vi "SET_play.vi"() -> ()   [LabVIEW 2018]
uses:
  Ctrl/SET_1111.ctl
  Ctrl/SET_1112.ctl
  Ctrl/SET_1113.ctl
  Ctrl/SET_1121.ctl
  Ctrl/SET_1122.ctl
  Ctrl/SET_1123.ctl
  Ctrl/SET_1131.ctl
  Ctrl/SET_1132.ctl
  Ctrl/SET_1133.ctl
  Ctrl/SET_1211.ctl
  Ctrl/SET_1212.ctl
  Ctrl/SET_1213.ctl
  Ctrl/SET_1221.ctl
  Ctrl/SET_1222.ctl
  Ctrl/SET_1223.ctl
  Ctrl/SET_1231.ctl
  Ctrl/SET_1232.ctl
  Ctrl/SET_1233.ctl
  Ctrl/SET_1311.ctl
  Ctrl/SET_1312.ctl
  Ctrl/SET_1313.ctl
  Ctrl/SET_1321.ctl
  Ctrl/SET_1322.ctl
  Ctrl/SET_1323.ctl
  Ctrl/SET_1331.ctl
  Ctrl/SET_1332.ctl
  Ctrl/SET_1333.ctl
  Ctrl/SET_2111.ctl
  Ctrl/SET_2112.ctl
  Ctrl/SET_2113.ctl
  Ctrl/SET_2121.ctl
  Ctrl/SET_2122.ctl
  Ctrl/SET_2123.ctl
  Ctrl/SET_2131.ctl
  Ctrl/SET_2132.ctl
  Ctrl/SET_2133.ctl
  Ctrl/SET_2211.ctl
  Ctrl/SET_2212.ctl
  Ctrl/SET_2213.ctl
  Ctrl/SET_2221.ctl
  Ctrl/SET_2222.ctl
  Ctrl/SET_2223.ctl
  Ctrl/SET_2231.ctl
  Ctrl/SET_2232.ctl
  Ctrl/SET_2233.ctl
  Ctrl/SET_2311.ctl
  Ctrl/SET_2312.ctl
  Ctrl/SET_2313.ctl
  Ctrl/SET_2321.ctl
  Ctrl/SET_2322.ctl
  Ctrl/SET_2323.ctl
  Ctrl/SET_2331.ctl
  Ctrl/SET_2332.ctl
  Ctrl/SET_2333.ctl
  Ctrl/SET_3111.ctl
  Ctrl/SET_3112.ctl
  Ctrl/SET_3113.ctl
  Ctrl/SET_3121.ctl
  Ctrl/SET_3122.ctl
  Ctrl/SET_3123.ctl
  Ctrl/SET_3131.ctl
  Ctrl/SET_3132.ctl
  Ctrl/SET_3133.ctl
  Ctrl/SET_3211.ctl
  Ctrl/SET_3212.ctl
  Ctrl/SET_3213.ctl
  Ctrl/SET_3221.ctl
  Ctrl/SET_3222.ctl
  Ctrl/SET_3223.ctl
  Ctrl/SET_3231.ctl
  Ctrl/SET_3232.ctl
  Ctrl/SET_3233.ctl
  Ctrl/SET_3311.ctl
  Ctrl/SET_3312.ctl
  Ctrl/SET_3313.ctl
  Ctrl/SET_3321.ctl
  Ctrl/SET_3322.ctl
  Ctrl/SET_3323.ctl
  Ctrl/SET_3331.ctl
  Ctrl/SET_3332.ctl
  Ctrl/SET_3333.ctl
  Ctrl/Button_turn.ctl
  Ctrl/Delay_time_display.ctl
  Ctrl/Color_box.ctl
  <vilib>/Utility/miscctls.llb/LVBoundsTypeDef.ctl
  <vilib>/Utility/miscctls.llb/LVPositionTypeDef.ctl
  Ctrl/Menu.ctl
  8331993e-770e-4ab0-80c5-ef35aa114950.vi
  2b4e26d8-541c-4eaa-9e7c-42fc4059c27e.vi
panel:
  out "Hint_idx":u8
  out "Matching_idx":i32[][](array[numeric])
  out "Total_ID":i32[](array[numeric])
  out "Count_shuffle":i32=12
  out "ID_select_cards":i32[](array[numeric])
  out "idx_select_cards":i32[](array[numeric])
  out "Start_time(ms)":u32
  out "Turn":bool
  out "POS_of_cards":T1[](array[typedef])
  out "main_cards":refnum<vi>[](array[refnum])
  out "Ref_turn_btn":refnum<vi>[](array[refnum])
  out "Time_turn(ms)":u32
  out "Time_disadvantage(ms)":u32
  out "Ref_card_shuffle":refnum<vi>[](array[refnum])
  out "Tab_bounds":T2 caption="경계"
  out "Ref_card":refnum<vi>[](array[refnum])
  out "Tab_ctrl":enum32{"페이지 1", "페이지 2", "페이지 3"}(tab)
  in  "exit_program":bool
  out "num_SET":u8
  out "num_remain_cards":u8
  out "Delay_2P":T3 scale=0.0..1.0
  in  "Turn_2P":T4
  out "Delay_1P":T3 scale=0.0..1.0
  in  "Turn_1P":T4
  in  "불리언 81":T5
  in  "불리언 80":T6
  in  "불리언 79":T7
  in  "불리언 78":T8
  in  "불리언 77":T9
  in  "불리언 76":T10
  in  "불리언 75":T11
  in  "불리언 74":T12
  in  "불리언 73":T13
  in  "불리언 72":T14
  in  "불리언 71":T15
  in  "불리언 70":T16
  in  "불리언 69":T17
  in  "불리언 68":T18
  in  "불리언 67":T19
  in  "불리언 66":T20
  in  "불리언 65":T21
  in  "불리언 64":T22
  in  "불리언 63":T23
  in  "불리언 62":T24
  in  "불리언 61":T25
  in  "불리언 60":T26
  in  "불리언 59":T27
  in  "불리언 58":T28
  in  "불리언 57":T29
  in  "불리언 56":T30
  in  "불리언 55":T31
  in  "불리언 54":T32
  in  "불리언 53":T33
  in  "불리언 52":T34
  in  "불리언 51":T35
  in  "불리언 50":T36
  in  "불리언 49":T37
  in  "불리언 48":T38
  in  "불리언 47":T39
  in  "불리언 46":T40
  in  "불리언 45":T41
  in  "불리언 44":T42
  in  "불리언 43":T43
  in  "불리언 42":T44
  in  "불리언 41":T45
  in  "불리언 40":T46
  in  "불리언 39":T47
  in  "불리언 38":T48
  in  "불리언 37":T49
  in  "불리언 36":T50
  in  "불리언 35":T51
  in  "불리언 34":T52
  in  "불리언 33":T53
  in  "불리언 32":T54
  in  "불리언 31":T55
  in  "불리언 30":T56
  in  "불리언 29":T57
  in  "불리언 28":T58
  in  "불리언 27":T59
  in  "불리언 26":T60
  in  "불리언 25":T61
  in  "불리언 24":T62
  in  "불리언 23":T63
  in  "불리언 22":T64
  in  "불리언 21":T65
  in  "불리언 20":T66
  in  "불리언 19":T67
  in  "불리언 18":T68
  in  "불리언 17":T69
  in  "불리언 16":T70
  in  "불리언 15":T71
  in  "불리언 14":T72
  in  "불리언 13":T73
  in  "불리언 12":T74
  in  "불리언 11":T75
  in  "불리언 10":T76
  in  "불리언 9":T77
  in  "불리언 8":T78
  in  "불리언 7":T79
  in  "불리언 6":T80
  in  "불리언 5":T81
  in  "불리언 4":T82
  in  "불리언 3":T83
  in  "불리언 2":T84
  in  "불리언":T85
  out "Color_box_1P":T86
  out "Color_box_2P":T86
  in  "Button_start":bool
  out "Score_1P":i8
  out "Score_2P":i8
  in  "Btn_hint":bool
  # "1P\nScore"
  # "2P\nScore"
  # "남은\n카드"
  # "SET\n개수"
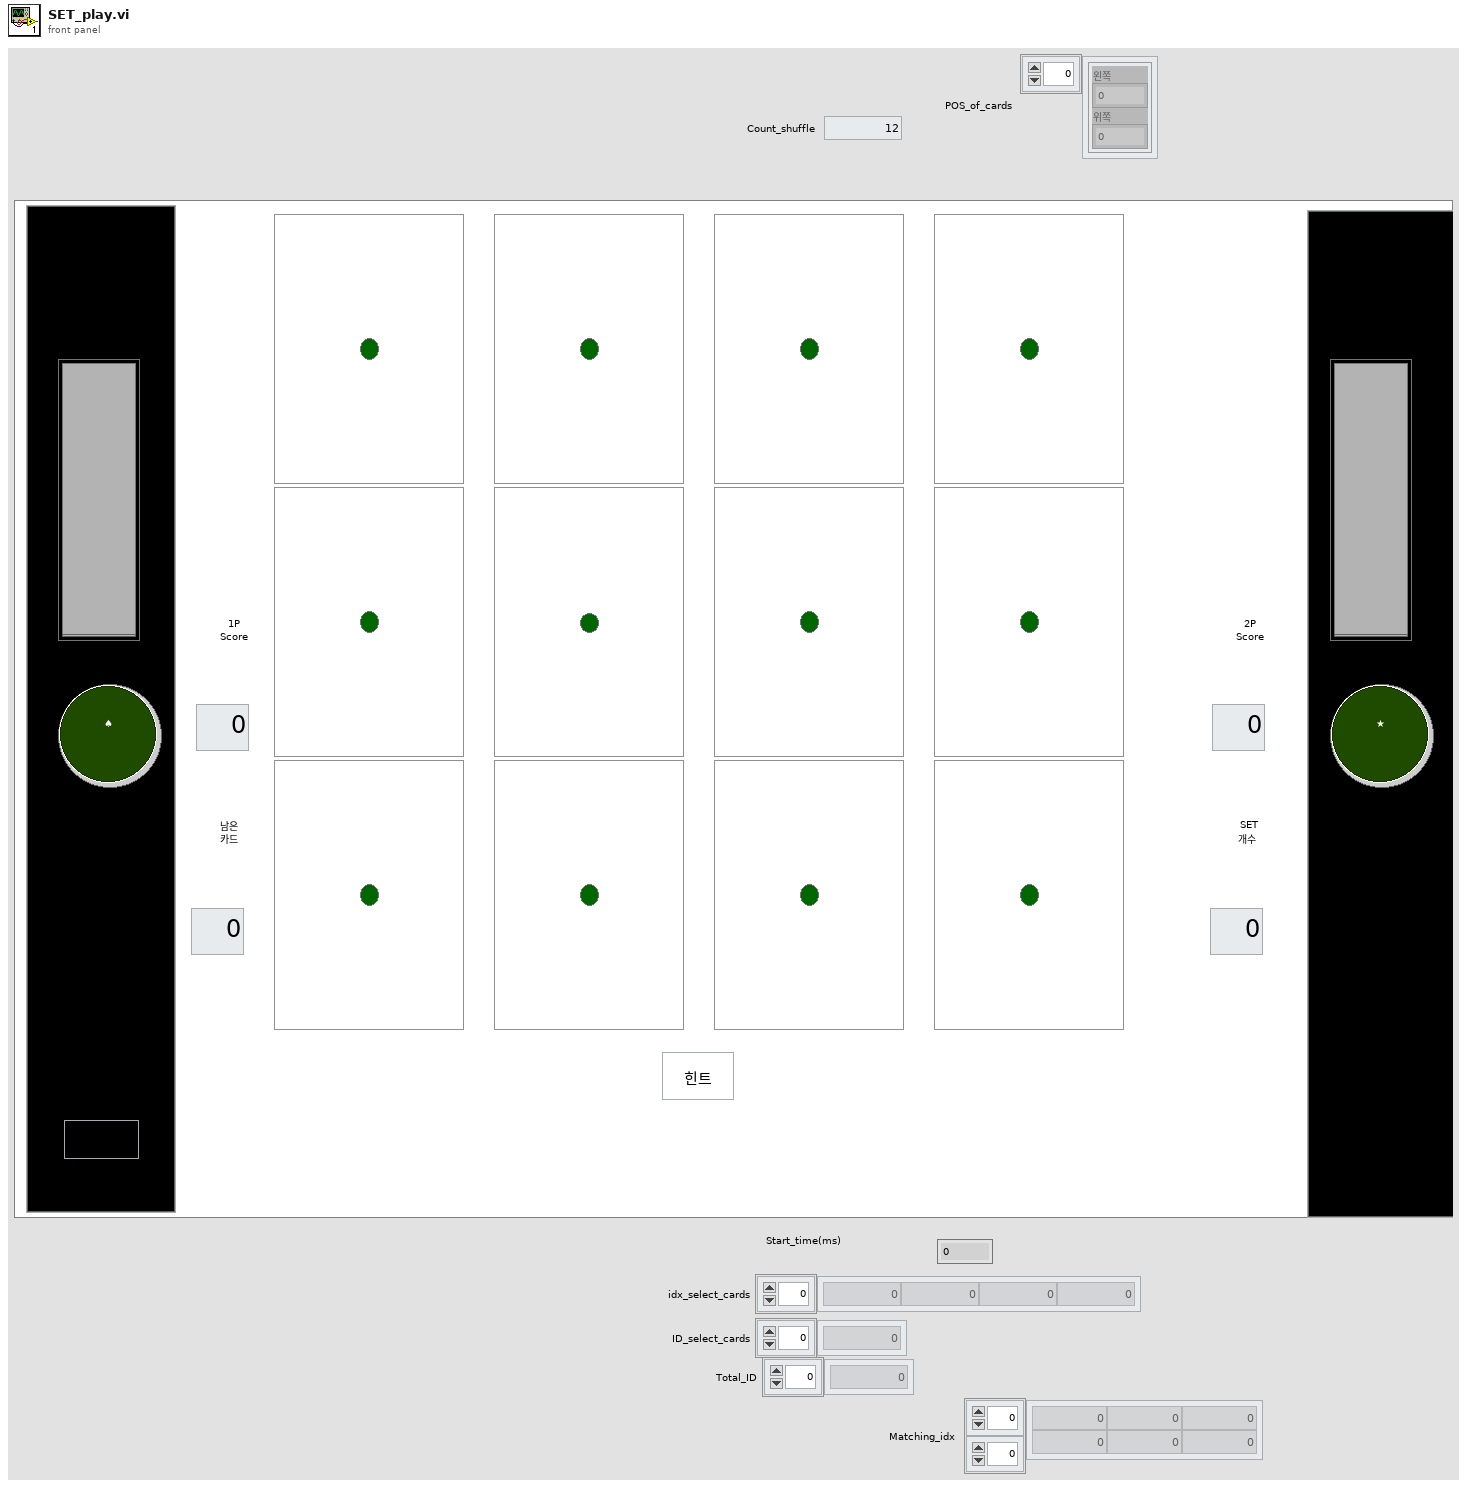
[diagram p1: front panel]
types:
  T1 = typedef "LVPositionTypeDef.ctl" = cluster{"Left":i32, "Top":i32}
  T2 = typedef "LVBoundsTypeDef.ctl" = cluster{"Width":u32, "Height":u32}
  T3 = typedef "Delay_time_display.ctl" = dbl
  T4 = typedef "Button_turn.ctl" = bool
  T5 = typedef "SET_3333.ctl" = bool
  T6 = typedef "SET_3332.ctl" = bool
  T7 = typedef "SET_3331.ctl" = bool
  T8 = typedef "SET_3323.ctl" = bool
  T9 = typedef "SET_3322.ctl" = bool
  T10 = typedef "SET_3321.ctl" = bool
  T11 = typedef "SET_3313.ctl" = bool
  T12 = typedef "SET_3312.ctl" = bool
  T13 = typedef "SET_3311.ctl" = bool
  T14 = typedef "SET_3233.ctl" = bool
  T15 = typedef "SET_3232.ctl" = bool
  T16 = typedef "SET_3231.ctl" = bool
  T17 = typedef "SET_3223.ctl" = bool
  T18 = typedef "SET_3222.ctl" = bool
  T19 = typedef "SET_3221.ctl" = bool
  T20 = typedef "SET_3213.ctl" = bool
  T21 = typedef "SET_3212.ctl" = bool
  T22 = typedef "SET_3211.ctl" = bool
  T23 = typedef "SET_3133.ctl" = bool
  T24 = typedef "SET_3132.ctl" = bool
  T25 = typedef "SET_3131.ctl" = bool
  T26 = typedef "SET_3123.ctl" = bool
  T27 = typedef "SET_3122.ctl" = bool
  T28 = typedef "SET_3121.ctl" = bool
  T29 = typedef "SET_3113.ctl" = bool
  T30 = typedef "SET_3112.ctl" = bool
  T31 = typedef "SET_3111.ctl" = bool
  T32 = typedef "SET_2333.ctl" = bool
  T33 = typedef "SET_2332.ctl" = bool
  T34 = typedef "SET_2331.ctl" = bool
  T35 = typedef "SET_2323.ctl" = bool
  T36 = typedef "SET_2322.ctl" = bool
  T37 = typedef "SET_2321.ctl" = bool
  T38 = typedef "SET_2313.ctl" = bool
  T39 = typedef "SET_2312.ctl" = bool
  T40 = typedef "SET_2311.ctl" = bool
  T41 = typedef "SET_2233.ctl" = bool
  T42 = typedef "SET_2232.ctl" = bool
  T43 = typedef "SET_2231.ctl" = bool
  T44 = typedef "SET_2223.ctl" = bool
  T45 = typedef "SET_2222.ctl" = bool
  T46 = typedef "SET_2221.ctl" = bool
  T47 = typedef "SET_2213.ctl" = bool
  T48 = typedef "SET_2212.ctl" = bool
  T49 = typedef "SET_2211.ctl" = bool
  T50 = typedef "SET_2133.ctl" = bool
  T51 = typedef "SET_2132.ctl" = bool
  T52 = typedef "SET_2131.ctl" = bool
  T53 = typedef "SET_2123.ctl" = bool
  T54 = typedef "SET_2122.ctl" = bool
  T55 = typedef "SET_2121.ctl" = bool
  T56 = typedef "SET_2113.ctl" = bool
  T57 = typedef "SET_2112.ctl" = bool
  T58 = typedef "SET_2111.ctl" = bool
  T59 = typedef "SET_1333.ctl" = bool
  T60 = typedef "SET_1332.ctl" = bool
  T61 = typedef "SET_1331.ctl" = bool
  T62 = typedef "SET_1323.ctl" = bool
  T63 = typedef "SET_1322.ctl" = bool
  T64 = typedef "SET_1321.ctl" = bool
  T65 = typedef "SET_1313.ctl" = bool
  T66 = typedef "SET_1312.ctl" = bool
  T67 = typedef "SET_1311.ctl" = bool
  T68 = typedef "SET_1233.ctl" = bool
  T69 = typedef "SET_1232.ctl" = bool
  T70 = typedef "SET_1231.ctl" = bool
  T71 = typedef "SET_1223.ctl" = bool
  T72 = typedef "SET_1222.ctl" = bool
  T73 = typedef "SET_1221.ctl" = bool
  T74 = typedef "SET_1213.ctl" = bool
  T75 = typedef "SET_1212.ctl" = bool
  T76 = typedef "SET_1211.ctl" = bool
  T77 = typedef "SET_1133.ctl" = bool
  T78 = typedef "SET_1132.ctl" = bool
  T79 = typedef "SET_1131.ctl" = bool
  T80 = typedef "SET_1123.ctl" = bool
  T81 = typedef "SET_1122.ctl" = bool
  T82 = typedef "SET_1121.ctl" = bool
  T83 = typedef "SET_1113.ctl" = bool
  T84 = typedef "SET_1112.ctl" = bool
  T85 = typedef "SET_1111.ctl" = bool
  T86 = typedef "Color_box.ctl" = u32
  T87 = typedef "Menu.ctl" = enum16{"Select turn", "Initialization", "Make variable_1", "Make variable_2", "Ready game", "Choose cards", "Penalty", "Card matching", "Card checking", "Finish game", "Shuffle cards", "Hint"}
  T88 = enum8{"Enabled", "Disabled", "Disabled and Grayed Out"}
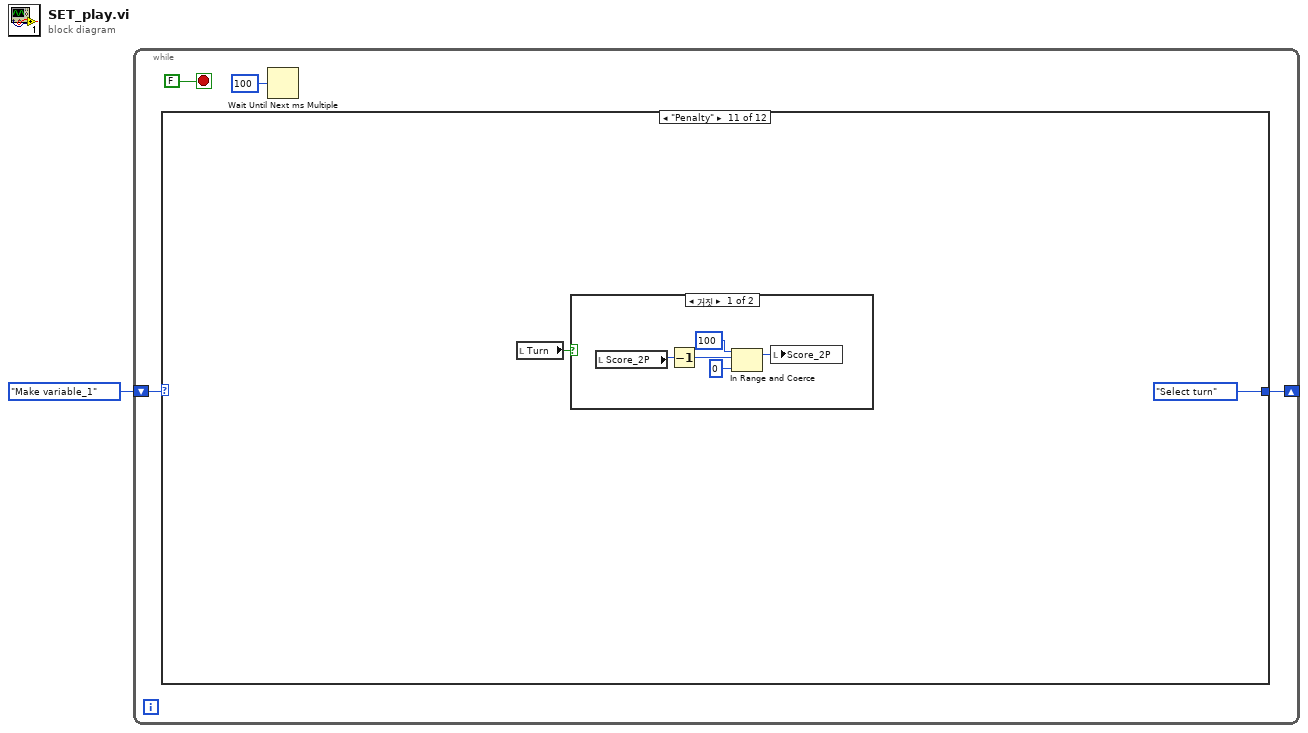
[diagram p0: block diagram]
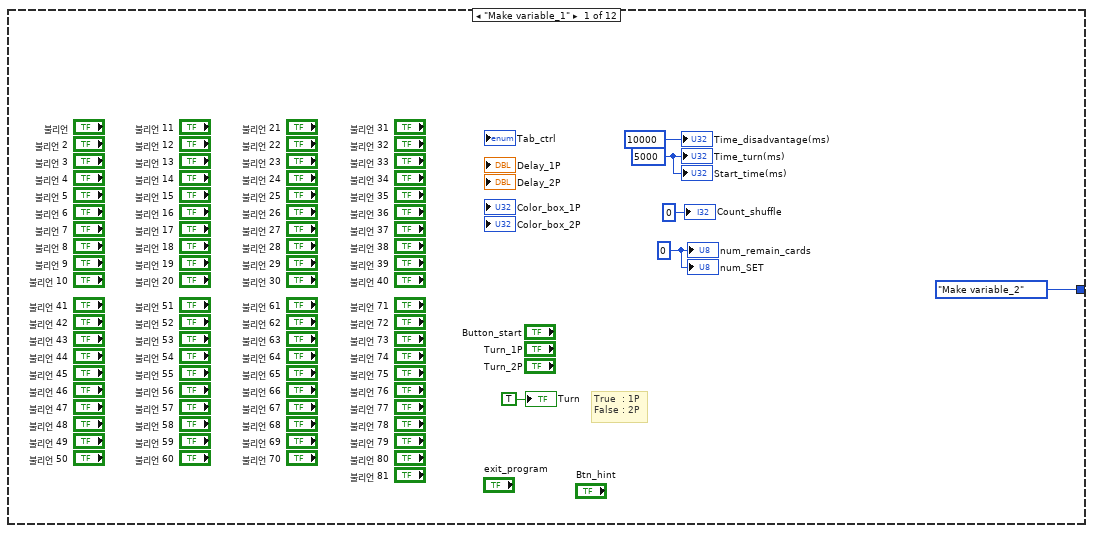
[diagram p2: hidden frame]
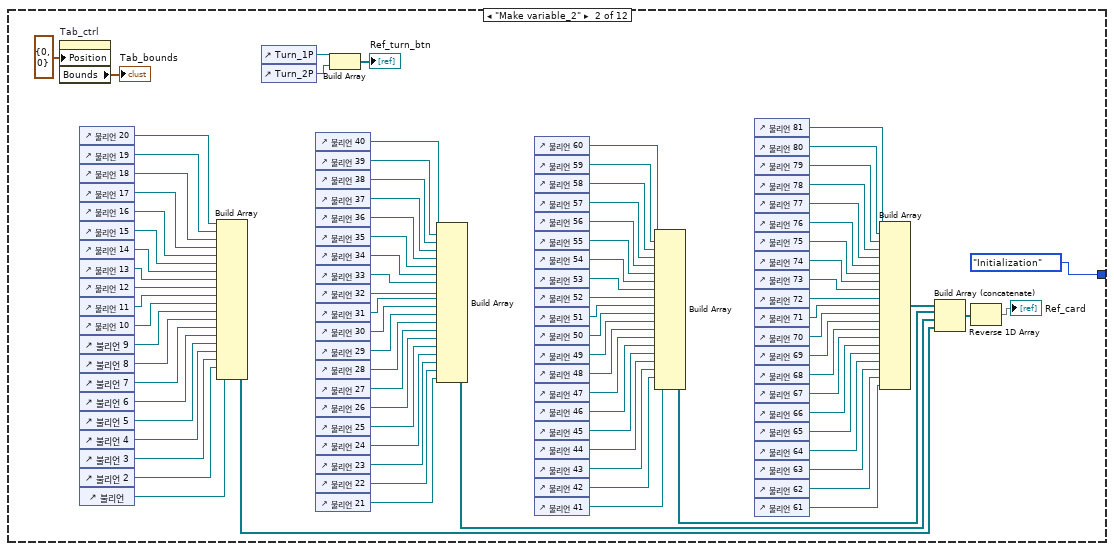
[diagram p3: hidden frame]
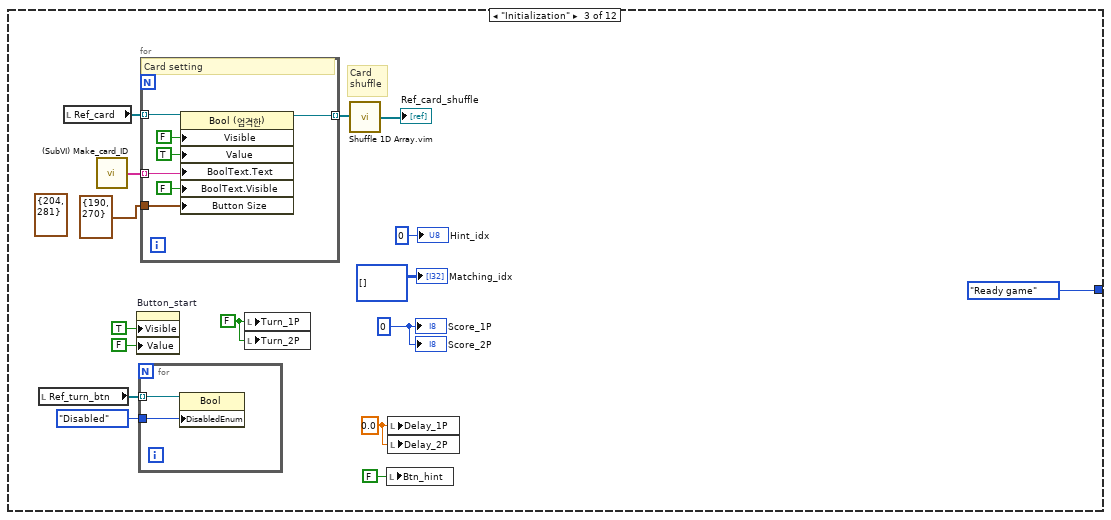
[diagram p4: hidden frame]
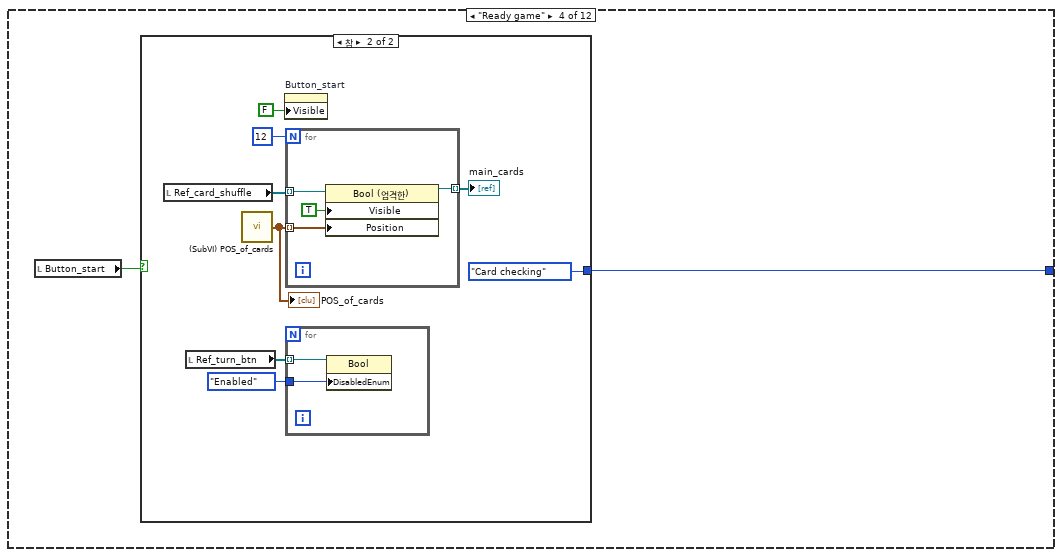
[diagram p5: hidden frame]
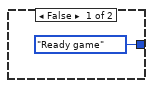
[diagram p6: hidden frame]
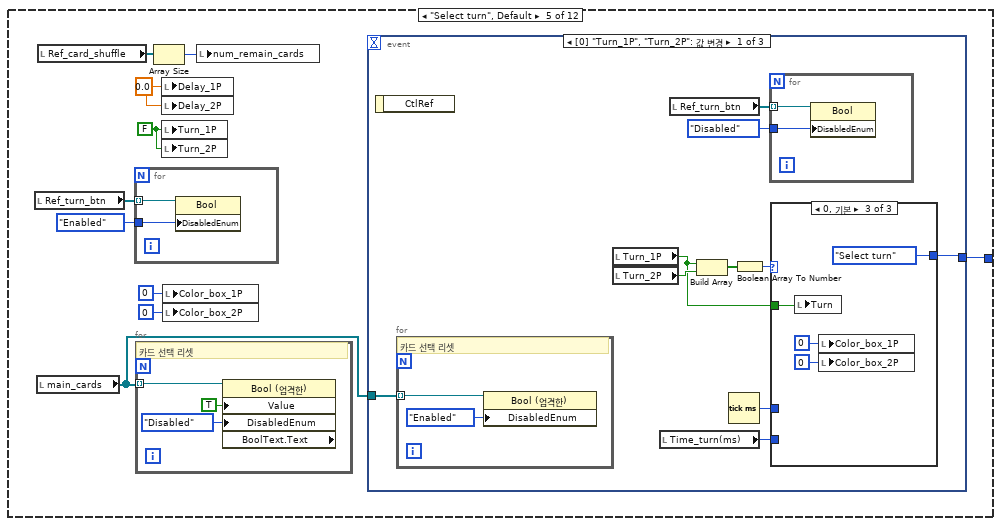
[diagram p7: hidden frame]
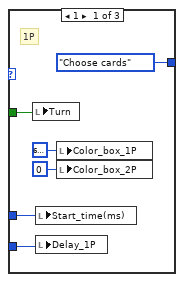
[diagram p8: hidden frame]
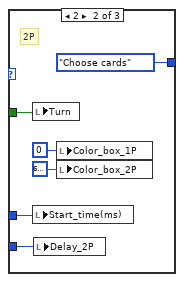
[diagram p9: hidden frame]
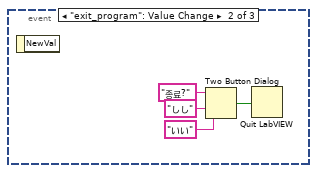
[diagram p10: hidden frame]
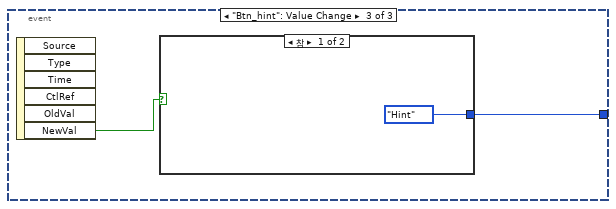
[diagram p11: hidden frame]
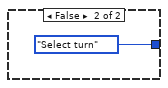
[diagram p12: hidden frame]
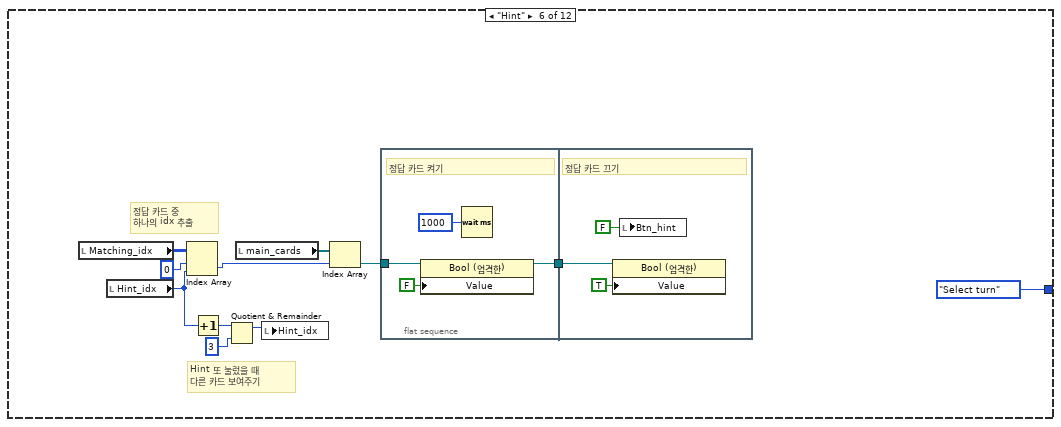
[diagram p13: hidden frame]
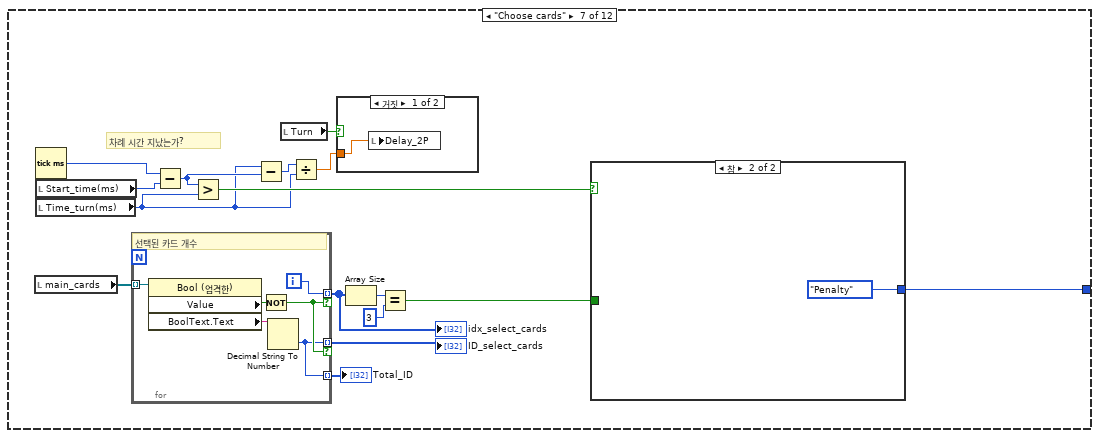
[diagram p14: hidden frame]
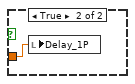
[diagram p15: hidden frame]
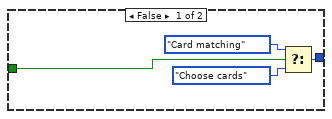
[diagram p16: hidden frame]
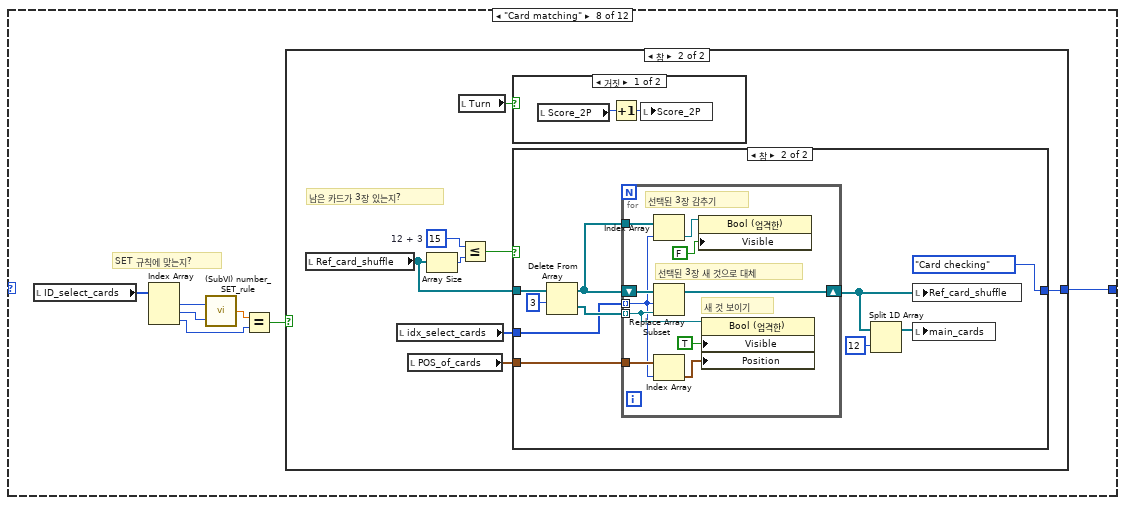
[diagram p17: hidden frame]
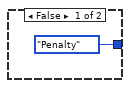
[diagram p18: hidden frame]
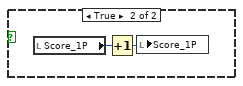
[diagram p19: hidden frame]
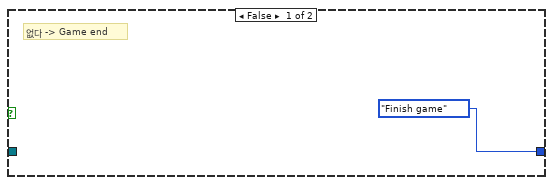
[diagram p20: hidden frame]
diagram:
  n1 = while {
    shift-right: [w3] -> _
    shift-left: Menu."Make variable_1" ("열거형") -> [w4]
    stop <- FALSE stop-if-true
    n2 = case shown="\"Penalty\"" w4 {
      tunnel: [Menu."Make variable_2" ("열거형") Menu."Initialization" ("열거형") Menu."Ready game" ("열거형") w131 w156 Menu."Select turn" ("열거형") w225 w247 w294 w306 Menu."Select turn" ("열거형") Menu."Make variable_1" ("열거형")] -> w3
      frame "Make variable_1" {
        w6 = u8 0 ("num_remain_cards")
        w8 = u32 5000 ("Time_turn(ms)")
        # "True  : 1P\nFalse : 2P"
        "Time_disadvantage(ms)" <- u32 10000 ("Time_disadvantage")
        "Time_turn(ms)" <- w8
        "Turn" <- TRUE ("Turn")
        "Start_time(ms)" <- w8
        "Count_shuffle" <- 0 ("Count_shuffle")
        "num_remain_cards" <- w6
        "num_SET" <- w6
      }
      frame "Make variable_2" {
        n3 = property on="Tab_ctrl" class="TabCtl (엄격한)"("Position"=T1 {"Left"=0, "Top"=0} ("위치")) -> ("Bounds"=→"Tab_bounds":T2)  [unwired: 2 in, 2 out]
        n4 = control-ref of="불리언 20"() -> (w25:refnum<vi>)
        n5 = control-ref of="불리언 19"() -> (w26:refnum<vi>)
        n6 = control-ref of="불리언 18"() -> (w27:refnum<vi>)
        n7 = control-ref of="불리언 17"() -> (w28:refnum<vi>)
        n8 = control-ref of="불리언 16"() -> (w29:refnum<vi>)
        n9 = control-ref of="불리언 15"() -> (w30:refnum<vi>)
        n10 = control-ref of="불리언 14"() -> (w31:refnum<vi>)
        n11 = control-ref of="불리언 13"() -> (w32:refnum<vi>)
        n12 = control-ref of="불리언 12"() -> (w33:refnum<vi>)
        n13 = control-ref of="불리언 11"() -> (w34:refnum<vi>)
        n14 = control-ref of="불리언 10"() -> (w35:refnum<vi>)
        n15 = control-ref of="불리언 9"() -> (w36:refnum<vi>)
        n16 = control-ref of="불리언 8"() -> (w37:refnum<vi>)
        n17 = control-ref of="불리언 7"() -> (w38:refnum<vi>)
        n18 = control-ref of="불리언 6"() -> (w39:refnum<vi>)
        n19 = control-ref of="불리언 5"() -> (w40:refnum<vi>)
        n20 = control-ref of="불리언 4"() -> (w41:refnum<vi>)
        n21 = control-ref of="불리언 3"() -> (w42:refnum<vi>)
        n22 = control-ref of="불리언 2"() -> (w43:refnum<vi>)
        n23 = control-ref of="불리언"() -> (w44:refnum<vi>)
        n24 = Build Array(w25, w26, w27, w28, w29, w30, w31, w32, w33, w34, w35, w36, w37, w38, w39, w40, w41, w42, w43, w44) -> (w20:refnum<vi>[])
        n25 = control-ref of="Turn_1P"() -> (w13:refnum<vi>)
        n26 = control-ref of="Turn_2P"() -> (w14:refnum<vi>)
        n27 = control-ref of="불리언 40"() -> (w45:refnum<vi>)
        n28 = control-ref of="불리언 39"() -> (w46:refnum<vi>)
        n29 = control-ref of="불리언 38"() -> (w47:refnum<vi>)
        n30 = control-ref of="불리언 37"() -> (w48:refnum<vi>)
        n31 = control-ref of="불리언 36"() -> (w49:refnum<vi>)
        n32 = control-ref of="불리언 35"() -> (w50:refnum<vi>)
        n33 = control-ref of="불리언 34"() -> (w51:refnum<vi>)
        n34 = control-ref of="불리언 33"() -> (w52:refnum<vi>)
        n35 = control-ref of="불리언 32"() -> (w53:refnum<vi>)
        n36 = control-ref of="불리언 31"() -> (w54:refnum<vi>)
        n37 = control-ref of="불리언 30"() -> (w55:refnum<vi>)
        n38 = control-ref of="불리언 29"() -> (w56:refnum<vi>)
        n39 = control-ref of="불리언 28"() -> (w57:refnum<vi>)
        n40 = control-ref of="불리언 27"() -> (w58:refnum<vi>)
        n41 = control-ref of="불리언 26"() -> (w59:refnum<vi>)
        n42 = control-ref of="불리언 25"() -> (w60:refnum<vi>)
        n43 = control-ref of="불리언 24"() -> (w61:refnum<vi>)
        n44 = control-ref of="불리언 23"() -> (w62:refnum<vi>)
        n45 = control-ref of="불리언 22"() -> (w63:refnum<vi>)
        n46 = control-ref of="불리언 21"() -> (w64:refnum<vi>)
        n47 = Build Array(w13, w14) -> (→"Ref_turn_btn":refnum<vi>[])
        n48 = Build Array(w45, w46, w47, w48, w49, w50, w51, w52, w53, w54, w55, w56, w57, w58, w59, w60, w61, w62, w63, w64) -> (w21:refnum<vi>[])
        n49 = control-ref of="불리언 60"() -> (w65:refnum<vi>)
        n50 = control-ref of="불리언 59"() -> (w66:refnum<vi>)
        n51 = control-ref of="불리언 58"() -> (w67:refnum<vi>)
        n52 = control-ref of="불리언 57"() -> (w68:refnum<vi>)
        n53 = control-ref of="불리언 56"() -> (w69:refnum<vi>)
        n54 = control-ref of="불리언 55"() -> (w70:refnum<vi>)
        n55 = control-ref of="불리언 54"() -> (w71:refnum<vi>)
        n56 = control-ref of="불리언 53"() -> (w72:refnum<vi>)
        n57 = control-ref of="불리언 52"() -> (w73:refnum<vi>)
        n58 = control-ref of="불리언 51"() -> (w74:refnum<vi>)
        n59 = control-ref of="불리언 50"() -> (w75:refnum<vi>)
        n60 = control-ref of="불리언 49"() -> (w76:refnum<vi>)
        n61 = control-ref of="불리언 48"() -> (w77:refnum<vi>)
        n62 = control-ref of="불리언 47"() -> (w78:refnum<vi>)
        n63 = control-ref of="불리언 46"() -> (w79:refnum<vi>)
        n64 = control-ref of="불리언 45"() -> (w80:refnum<vi>)
        n65 = control-ref of="불리언 44"() -> (w81:refnum<vi>)
        n66 = control-ref of="불리언 43"() -> (w82:refnum<vi>)
        n67 = control-ref of="불리언 42"() -> (w83:refnum<vi>)
        n68 = control-ref of="불리언 41"() -> (w84:refnum<vi>)
        n69 = Build Array(w65, w66, w67, w68, w69, w70, w71, w72, w73, w74, w75, w76, w77, w78, w79, w80, w81, w82, w83, w84) -> (w22:refnum<vi>[])
        n70 = control-ref of="불리언 81"() -> (w24:refnum<vi>)
        n71 = control-ref of="불리언 80"() -> (w85:refnum<vi>)
        n72 = control-ref of="불리언 79"() -> (w86:refnum<vi>)
        n73 = control-ref of="불리언 78"() -> (w87:refnum<vi>)
        n74 = control-ref of="불리언 77"() -> (w88:refnum<vi>)
        n75 = control-ref of="불리언 76"() -> (w89:refnum<vi>)
        n76 = control-ref of="불리언 75"() -> (w90:refnum<vi>)
        n77 = control-ref of="불리언 74"() -> (w91:refnum<vi>)
        n78 = control-ref of="불리언 73"() -> (w92:refnum<vi>)
        n79 = control-ref of="불리언 72"() -> (w93:refnum<vi>)
        n80 = control-ref of="불리언 71"() -> (w94:refnum<vi>)
        n81 = control-ref of="불리언 70"() -> (w95:refnum<vi>)
        n82 = control-ref of="불리언 69"() -> (w96:refnum<vi>)
        n83 = control-ref of="불리언 68"() -> (w97:refnum<vi>)
        n84 = control-ref of="불리언 67"() -> (w98:refnum<vi>)
        n85 = control-ref of="불리언 66"() -> (w99:refnum<vi>)
        n86 = control-ref of="불리언 65"() -> (w100:refnum<vi>)
        n87 = control-ref of="불리언 64"() -> (w101:refnum<vi>)
        n88 = control-ref of="불리언 63"() -> (w102:refnum<vi>)
        n89 = control-ref of="불리언 62"() -> (w103:refnum<vi>)
        n90 = control-ref of="불리언 61"() -> (w104:refnum<vi>)
        n91 = Build Array(w24, w85, w86, w87, w88, w89, w90, w91, w92, w93, w94, w95, w96, w97, w98, w99, w100, w101, w102, w103, w104) -> (w23:refnum<vi>[])
        n92 = Build Array (concatenate)(w23, w22, w21, w20) -> (w19:refnum<vi>[])
        n93 = Reverse 1D Array(array=w19) -> (reversed array=→"Ref_card":refnum<vi>[])
      }
      frame "Initialization" {
        w105 = i8 0 ("Score_1P")
        (unwired) T2 {"Width"=204, "Height"=281} ("버튼 크기")
        w110 = T3 0.0 ("Delay_1P")
        w113 = T4 FALSE ("Turn_1P")
        # "Card \nshuffle"
        n94 = local read "Ref_turn_btn"() -> (w114:refnum<vi>[])
        n95 = local read "Ref_card"() -> (w120:refnum<vi>[])
        n96 = call "(SubVI) Make_card_ID.vi"() -> ("Card_ID"=w119:string[])
        n97 = property on="Button_start" class="Bool (엄격한)"("Visible"=TRUE ("보이기"), "Value"=FALSE ("Button_start")) -> ()  [unwired: 2 in, 2 out]
        n98 = for {
          tunnel: T88."Disabled" ("비활성화") -> [w122]
          tunnel: w114 -> [w121] mode=indexing
          n99 = property class="Bool"(reference=w121, "DisabledEnum"=w122) -> ()  [unwired: 1 in, 2 out]
        }
        n100 = for {
          tunnel: w120 -> [w129] mode=indexing
          tunnel: w119 -> [w125] mode=indexing
          tunnel: [w124] -> w118 mode=indexing
          tunnel: T2 {"Width"=190, "Height"=270} ("버튼 크기") -> [w123]
          # "Card setting"
          n101 = property class="Bool (엄격한)"(reference=w129, "Visible"=FALSE ("보이기"), "Value"=T85 TRUE ("값"), "BoolText.Text"=w125, "BoolText.Visible"=FALSE ("불리언 텍스트.보이기"), "Button Size"=w123) -> (reference out=w124:refnum<vi>)  [unwired: 1 in, 1 out]
        }
        n102 = local write "Turn_1P"(w113) -> ()
        n103 = local write "Turn_2P"(w113) -> ()
        n104 = call "Shuffle 1D Array.vim"("array"=w118) -> ("shuffled array"=→"Ref_card_shuffle":refnum<vi>[])  [unwired: 4 in]
        n105 = local write "Btn_hint"(FALSE ("Btn_hint")) -> ()
        n106 = local write "Delay_1P"(w110) -> ()
        n107 = local write "Delay_2P"(w110) -> ()
        "Score_1P" <- w105
        "Score_2P" <- w105
        "Matching_idx" <- i32[][] [] ("Matching_idx")
        "Hint_idx" <- u8 0 ("Hint_idx")
      }
      frame "Ready game" {
        n108 = local read "Button_start"() -> (w130:bool)
        n109 = case shown="참" w130 {
          tunnel: [Menu."Ready game" ("열거형") Menu."Card checking" ("열거형")] -> w131
          frame False {
          }
          frame True {
            n110 = local read "Ref_card_shuffle"() -> (w138:refnum<vi>[])
            n111 = local read "Ref_turn_btn"() -> (w136:refnum<vi>[])
            n112 = call "(SubVI) POS_of_cards.vi"() -> ("POS_of_cards"=w139:T1[])
            "POS_of_cards" <- w139
            n113 = property on="Button_start" class="Bool (엄격한)"("Visible"=FALSE ("보이기")) -> ()  [unwired: 2 in, 2 out]
            n114 = for {
              N: 12 -> [_]
              tunnel: w138 -> [w146] mode=indexing
              tunnel: w139 -> [w144] mode=indexing
              tunnel: [w143] -> w133 mode=indexing
              n115 = property class="Bool (엄격한)"(reference=w146, "Visible"=TRUE ("보이기"), "Position"=w144) -> (reference out=w143:refnum<vi>)  [unwired: 1 in, 1 out]
            }
            "main_cards" <- w133
            n116 = for {
              tunnel: T88."Enabled" ("비활성화") -> [w142]
              tunnel: w136 -> [w141] mode=indexing
              n117 = property class="Bool"(reference=w141, "DisabledEnum"=w142) -> ()  [unwired: 1 in, 2 out]
            }
          }
        }
      }
      frame "Select turn", Default {
        w149 = T3 0.0 ("Delay_1P")
        w150 = T4 FALSE ("Turn_1P")
        n118 = local read "Ref_turn_btn"() -> (w151:refnum<vi>[])
        n119 = local read "main_cards"() -> (w155:refnum<vi>[])
        n120 = local read "Ref_card_shuffle"() -> (w147:refnum<vi>[])
        n121 = for {
          tunnel: T88."Enabled" ("비활성화") -> [w158]
          tunnel: w151 -> [w157] mode=indexing
          n122 = property class="Bool"(reference=w157, "DisabledEnum"=w158) -> ()  [unwired: 1 in, 2 out]
        }
        n123 = for {
          tunnel: w155 -> [w160] mode=indexing
          # "카드 선택 리셋"
          n124 = property class="Bool (엄격한)" props=["Value", "DisabledEnum", "BoolText", "Text"](reference=w160, "Value"=TRUE ("보이기"), "DisabledEnum"=T88."Disabled" ("비활성화")) -> ()  [unwired: 1 in, 3 out]
        }
        n125 = Array Size(array=w147) -> (size(s)=w148:i32)
        n126 = local write "Delay_1P"(w149) -> ()
        n127 = local write "Delay_2P"(w149) -> ()
        n128 = local write "Turn_1P"(w150) -> ()
        n129 = local write "Turn_2P"(w150) -> ()
        n130 = local write "Color_box_1P"(T86 0 ("Color_box_1P")) -> ()
        n131 = local write "Color_box_2P"(T86 0 ("Color_box_2P")) -> ()
        n132 = local write "num_remain_cards"(w148) -> ()
        n133 = event shown="[0] \"Turn_1P\", \"Turn_2P\": 값 변경" {
          selector: _ -> [_ _ _]
          dyn-events: _ -> [_ _ _]
          timeout: _ -> [_ _ _]
          tunnel: [w168 _ w196] -> w156
          tunnel: w155 -> [w163 _ _]
          event Value Change {
            n134 = event-data() -> ()  [unwired: 1 in, 1 out]
            n135 = for {
              tunnel: w163 -> [w172] mode=indexing
              # "카드 선택 리셋"
              n136 = property class="Bool (엄격한)"(reference=w172, "DisabledEnum"=T88."Enabled" ("비활성화")) -> ()  [unwired: 1 in, 2 out]
            }
            n137 = local read "Turn_1P"() -> (w167:T4)
            n138 = local read "Turn_2P"() -> (w171:T4)
            n139 = local read "Time_turn(ms)"() -> (w162:u32)
            n140 = local read "Ref_turn_btn"() -> (w170:refnum<vi>[])
            n141 = Build Array(w167, w171) -> (w166:T4[])
            n142 = Tick Count (ms)() -> (millisecond timer value=w164:u32)
            n143 = Boolean Array To Number(Boolean array=w166) -> (number=w165:u32)
            n144 = for {
              tunnel: T88."Disabled" ("비활성화") -> [w191]
              tunnel: w170 -> [w190] mode=indexing
              n145 = property class="Bool"(reference=w190, "DisabledEnum"=w191) -> ()  [unwired: 1 in, 2 out]
            }
            n146 = case shown="0, 기본" w165 {
              tunnel: [Menu."Choose cards" ("열거형") Menu."Choose cards" ("열거형") Menu."Select turn" ("열거형")] -> w168
              tunnel: w167 -> [w178 w184 w188]
              tunnel: w164 -> [w175 w181 _]
              tunnel: w162 -> [w174 w180 _]
              frame 1 {
                # "1P"
                n147 = local write "Turn"(w178) -> ()
                n148 = local write "Start_time(ms)"(w175) -> ()
                n149 = local write "Delay_1P"(w174) -> ()
                n150 = local write "Color_box_1P"(T86 6618880 ("Color_box_1P")) -> ()
                n151 = local write "Color_box_2P"(T86 0 ("Color_box_2P")) -> ()
              }
              frame 2 {
                # "2P"
                n152 = local write "Turn"(w184) -> ()
                n153 = local write "Start_time(ms)"(w181) -> ()
                n154 = local write "Delay_2P"(w180) -> ()
                n155 = local write "Color_box_1P"(T86 0 ("Color_box_1P")) -> ()
                n156 = local write "Color_box_2P"(T86 6618880 ("Color_box_2P")) -> ()
              }
              frame 0, Default {
                n157 = local write "Turn"(w188) -> ()
                n158 = local write "Color_box_1P"(T86 0 ("Color_box_1P")) -> ()
                n159 = local write "Color_box_2P"(T86 0 ("Color_box_2P")) -> ()
              }
            }
          }
          event "exit_program": Value Change {
            n160 = event-data() -> ()  [unwired: 1 in, 1 out]
            n161 = Two Button Dialog(message="종료?" ("메시지"), 1:"いい" ("거짓 버튼 이름(\"취소\")"), 2:"しし" ("참 버튼 이름(\"확인\")")) -> (T button?=w192:bool)
            n162 = Quit LabVIEW(quit? (T)=w192) -> ()
          }
          event "Btn_hint": Value Change {
            n163 = event-data() -> ("NewVal"=w197:bool)  [unwired: 1 in, 5 out]
            n164 = case shown="참" w197 {
              tunnel: [Menu."Hint" ("열거형") Menu."Select turn" ("열거형")] -> w196
              frame True {
              }
              frame False {
              }
            }
          }
        }
      }
      frame "Hint" {
        # "Hint 또 눌렀을 때 \n다른 카드 보여주기"
        # "정답 카드 중 \n하나의 idx 추출"
        n165 = local read "Matching_idx"() -> (w209:i32[][])
        n166 = local read "Hint_idx"() -> (w207:u8)
        n167 = Index Array(array=w209, index (row)=0 ("비활성화된 인덱스 (행)"), index (col)=w207) -> (element=w202:i32)
        n168 = Increment(x=w207) -> (x+1=w206:u8)
        n169 = Quotient & Remainder(x=w206, y=u8 3) -> (x-y*floor(x/y)=w204:u8)  [unwired: 1 out]
        n170 = local read "main_cards"() -> (w203:refnum<vi>[])
        n171 = local write "Hint_idx"(w204) -> ()
        n172 = Index Array(array=w203, index=w202) -> (element=w201:refnum<vi>)
        n173 = flat-sequence {
          tunnel: w201 -> [w213]
          tunnel: [w211] -> w200
          tunnel: w200 -> [w216]
          frame #0 {
            # "정답 카드 켜기"
            n174 = property class="Bool (엄격한)"(reference=w213, "Value"=FALSE ("보이기")) -> (reference out=w211:refnum<vi>)  [unwired: 1 in, 1 out]
            n175 = Wait (ms)(milliseconds to wait=u32 1000 ("대기 시간 (ms)")) -> ()  [unwired: 1 out]
          }
          frame #1 {
            # "정답 카드 끄기"
            n176 = property class="Bool (엄격한)"(reference=w216, "Value"=TRUE ("보이기")) -> ()  [unwired: 1 in, 2 out]
            n177 = local write "Btn_hint"(FALSE ("Btn_hint")) -> ()
          }
        }
      }
      frame "Choose cards" {
        # "차례 시간 지났는가?"
        n178 = local read "main_cards"() -> (w231:refnum<vi>[])
        n179 = Tick Count (ms)() -> (millisecond timer value=w232:u32)
        n180 = local read "Start_time(ms)"() -> (w233:u32)
        n181 = local read "Time_turn(ms)"() -> (w220:u32)
        n182 = for {
          tunnel: w231 -> [w246] mode=indexing
          tunnel: [w244] -> w230 mode=indexing if=w242
          tunnel: [w241] -> w227 mode=indexing if=w242
          tunnel: [w241] -> w218 mode=indexing
          i -> [w244]
          # "선택된 카드 개수"
          n183 = property class="Bool (엄격한)"(reference=w246) -> ("Value"=w245:T85, "BoolText.Text"=w243:string)  [unwired: 1 in, 2 out]
          n184 = Not(x=w245) -> (.not. x?=w242:T85)
          n185 = Decimal String To Number(string=w243) -> (number=w241:i32)  [unwired: 2 in, 1 out]
        }
        "idx_select_cards" <- w230
        "ID_select_cards" <- w227
        "Total_ID" <- w218
        n186 = Subtract(x=w232, y=w233) -> (x-y=w222:u32)
        n187 = Greater?(x=w222, y=w220) -> (0:w224:bool)
        n188 = Subtract(x=w220, y=w222) -> (x-y=w221:u32)
        n189 = local read "Turn"() -> (w223:bool)
        n190 = Divide(x=w221, y=w220) -> (x/y=w219:dbl)
        n191 = case shown="거짓" w223 {
          tunnel: w219 -> [w234 w235]
          frame False {
            n192 = local write "Delay_2P"(w234) -> ()
          }
          frame True {
            n193 = local write "Delay_1P"(w235) -> ()
          }
        }
        n194 = Array Size(array=w230) -> (size(s)=w229:i32)
        n195 = Equal?(x=w229, y=3) -> (x = y?=w226:bool)
        n196 = case shown="참" w224 {
          tunnel: w226 -> [w237 _]
          tunnel: [w236 Menu."Penalty" ("열거형")] -> w225
          frame False {
            n197 = Select(t=Menu."Card matching" ("열거형"), s=w237, f=Menu."Choose cards" ("열거형")) -> (s? t:f=w236:T87)
          }
          frame True {
          }
        }
      }
      frame "Card matching" {
        # "SET 규칙에 맞는지?"
        n198 = local read "ID_select_cards"() -> (w248:i32[])
        n199 = Index Array(array=w248) -> (element #1=w253:i32, element #2=w252:i32, element #3=w250:i32)  [unwired: 3 in]
        n200 = call "(SubVI) number_SET_rule.vi"("Input_2"=w252, "Input_1"=w253) -> ("Matching_number"=w251:dbl)
        n201 = Equal?(x=w251, y=w250) -> (x = y?=w249:bool)
        n202 = case shown="참" w249 {
          tunnel: [Menu."Penalty" ("열거형") w256] -> w247
          frame False {
          }
          frame True {
            w259 = 15  # 12 + 3
            # "남은 카드가 3장 있는지?"
            n203 = local read "Ref_card_shuffle"() -> (w260:refnum<vi>[])
            n204 = local read "idx_select_cards"() -> (w258:i32[])
            n205 = local read "POS_of_cards"() -> (w257:T1[])
            n206 = Array Size(array=w260) -> (size(s)=w261:i32)
            n207 = local read "Turn"() -> (w255:bool)
            n208 = Less Or Equal?(x=w259, y=w261) -> (x <= y?=w262:bool)
            n209 = case shown="거짓" w255 {
              frame False {
                n210 = local read "Score_2P"() -> (w263:i8)
                n211 = Increment(x=w263) -> (x+1=w264:i8)
                n212 = local write "Score_2P"(w264) -> ()
              }
              frame True {
                n213 = local read "Score_1P"() -> (w266:i8)
                n214 = Increment(x=w266) -> (x+1=w265:i8)
                n215 = local write "Score_1P"(w265) -> ()
              }
            }
            n216 = case shown="참" w262 {
              tunnel: w260 -> [_ w275]
              tunnel: w258 -> [_ w273]
              tunnel: w257 -> [_ w272]
              tunnel: [Menu."Finish game" ("열거형") Menu."Card checking" ("열거형")] -> w256
              frame False {
                # "없다 -> Game end"
              }
              frame True {
                n217 = Delete From Array(array=w275, length=3 ("길이")) -> (deleted portion=w276:refnum<vi>[], array with subset deleted=w274:refnum<vi>[])  [unwired: 1 in]
                n218 = for {
                  shift-right: [w286] -> w270
                  shift-left: w274 -> [w287]
                  tunnel: w276 -> [w281] mode=indexing
                  tunnel: w274 -> [w285]
                  tunnel: w273 -> [w279] mode=indexing
                  tunnel: w272 -> [w280]
                  # "새 것 보이기"
                  # "선택된 3장 새 것으로 대체"
                  # "선택된 3장 감추기"
                  n219 = Index Array(array=w285, index=w279) -> (element=w284:refnum<vi>)
                  n220 = Replace Array Subset(array=w287, new element=w281, index=w279) -> (w286:refnum<vi>[])
                  n221 = Index Array(array=w280, index=w279) -> (element=w278:T1)
                  n222 = property class="Bool (엄격한)"(reference=w284, "Visible"=FALSE ("보이기")) -> ()  [unwired: 1 in, 2 out]
                  n223 = property class="Bool (엄격한)"(reference=w281, "Visible"=TRUE ("보이기"), "Position"=w278) -> ()  [unwired: 1 in, 2 out]
                }
                n224 = Split 1D Array(array=w270, index=12 ("인덱스")) -> (first subarray=w268:refnum<vi>[])  [unwired: 1 out]
                n225 = local write "Ref_card_shuffle"(w270) -> ()
                n226 = local write "main_cards"(w268) -> ()
              }
            }
          }
        }
      }
      frame "Card checking" {
        # "Matching card 있음?"
        n227 = local read "main_cards"() -> (w297:refnum<vi>[])
        n228 = for {
          tunnel: w297 -> [w300] mode=indexing
          tunnel: [w298] -> w296 mode=indexing
          n229 = property class="Bool (엄격한)"(reference=w300) -> ("BoolText.Text"=w299:string)  [unwired: 1 in, 2 out]
          n230 = Decimal String To Number(string=w299) -> (number=w298:i32)  [unwired: 2 in, 1 out]
        }
        n231 = call "(SubVI) number_SET_rule_in_12_cards.vi"("array_ID"=w296) -> ("Matching_idx"=w288:i32[][])
        n232 = Array Size(array=w288) -> (size(s)=w290:i32[])
        n233 = local write "Matching_idx"(w288) -> ()
        n234 = Multiply Array Elements(1:w290) -> (0:w295:i32)
        n235 = Index Array(array=w290) -> (element=w289:i32)  [unwired: 1 in]
        n236 = Not Equal To 0?(x=w295) -> (x != 0?=w293:bool)
        n237 = local write "num_SET"(w289) -> ()
        n238 = Select(t=Menu."Select turn" ("열거형"), s=w293, f=Menu."Shuffle cards" ("열거형")) -> (s? t:f=w294:T87)
      }
      frame "Shuffle cards" {
        # "3회 섞고도 SET 규칙 안 나오면 \nfinish game"
        # "Counting shuffle"
        n239 = local read "main_cards"() -> (w305:refnum<vi>[])
        n240 = flat-sequence {
          tunnel: w304 -> [w318]
          tunnel: [w318] -> w302
          tunnel: [w317] -> w301
          frame #0 {
            # "Shuffle cards"
            n241 = local read "Ref_card_shuffle"() -> (w321:refnum<vi>[])
            n242 = call "Shuffle 1D Array.vim"("array"=w321) -> ("shuffled array"=w319:refnum<vi>[])  [unwired: 4 in]
            n243 = Split 1D Array(array=w319, index=12 ("인덱스")) -> (first subarray=w317:refnum<vi>[])  [unwired: 1 out]
            n244 = local write "Ref_card_shuffle"(w319) -> ()
            n245 = local write "main_cards"(w317) -> ()
          }
        }
        n246 = for {
          tunnel: w305 -> [w323] mode=indexing
          tunnel: [w322] -> w304
          # "원래 카드 감추기"
          n247 = property class="Bool (엄격한)"(reference=w323, "Visible"=FALSE ("보이기")) -> (error out=w322:errorcluster)  [unwired: 1 in, 1 out]
        }
        n248 = local read "POS_of_cards"() -> (w303:T1[])
        n249 = for {
          tunnel: w301 -> [w315] mode=indexing
          tunnel: w303 -> [w314] mode=indexing
          tunnel: w302 -> [w313]
          # "카드 재배치"
          n250 = property class="Bool (엄격한)"(reference=w315, error in=w313, "Visible"=TRUE ("보이기"), "Position"=w314) -> ()  [unwired: 2 out]
        }
        n251 = local read "Count_shuffle"() -> (w310:i32)
        n252 = Increment(x=w310) -> (x+1=w312:i32)
        n253 = local write "Count_shuffle"(w312) -> ()
        n254 = Greater Or Equal?(x=w312, y=3 ("인덱스")) -> (x >= y?=w311:bool)
        n255 = Select(t=Menu."Finish game" ("열거형"), s=w311, f=Menu."Card checking" ("열거형")) -> (s? t:f=w306:T87)
      }
      frame "Penalty" {
        n256 = local read "Turn"() -> (w325:bool)
        n257 = case shown="거짓" w325 {
          frame False {
            n258 = local read "Score_2P"() -> (w331:i8)
            n259 = Decrement(x=w331) -> (x-1=w330:i8)
            n260 = In Range and Coerce(upper limit=i8 100 ("상위 리미트"), x=w330, lower limit=i8 0 ("하위 리미트")) -> (coerced(x)=w329:i8)  [unwired: 1 out]
            n261 = local write "Score_2P"(w329) -> ()
          }
          frame True {
            n262 = local read "Score_1P"() -> (w336:i8)
            n263 = Decrement(x=w336) -> (x-1=w335:i8)
            n264 = In Range and Coerce(upper limit=i8 100 ("상위 리미트"), x=w335, lower limit=i8 0 ("하위 리미트")) -> (coerced(x)=w334:i8)  [unwired: 1 out]
            n265 = local write "Score_1P"(w334) -> ()
          }
        }
      }
      frame "Finish game" {
        n266 = Stop(stop? (T)=TRUE ("정지? (참)")) -> ()
      }
    }
    n267 = Wait Until Next ms Multiple(millisecond multiple=u32 100 ("ms 배수")) -> ()  [unwired: 1 out]
  }
